vi "[-50011] Instance Not Found.vi"(8 "error in (no error)":errorcluster, 11 "RegExp":string) -> (0 "error out":errorcluster)   [LabVIEW 2017, in "TagDB RefManager.lvlib"]
uses:
  TagDB RefManager.lvlib
  <userlib>/_NEVSTOP/TagDB/TagDB.lvlib
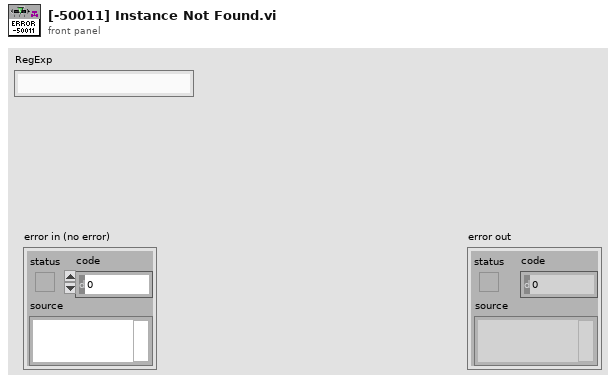
[diagram p1: front panel]
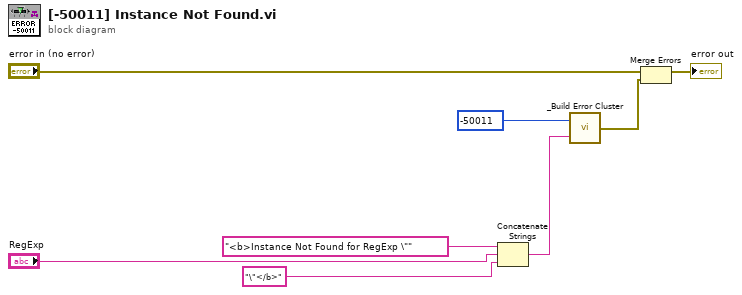
[diagram p0: block diagram]
diagram:
  n1 = Concatenate Strings("<b>Instance Not Found for RegExp \"" ("source"), "RegExp", "\"</b>" ("source")) -> (w1:string)
  n2 = call <userlib>:"_Build Error Cluster.vi"("String to Prepend to source (\"\")"=w1, "code"=-50011) -> ("error out"=w3:errorcluster)
  n3 = Merge Errors("error in (no error)", w3) -> (→"error out":errorcluster)
